vi "Render Recursive Partial with Wrong Key.vi"(8 "Error In":errorcluster) -> (0 "Error Out":errorcluster)   [LabVIEW 2018, in "Tests.lvlib" / "Render.lvlib"]
uses:
  Render.lvlib
  src/Toolkit/Data/Array/Array.lvclass
  D:/Users/cfield/Code/Field R&D Services/Labstache/src/Toolkit/Data/Datum/Datum.lvclass
  src/Toolkit/Data/Map/Map.lvclass
  src/Toolkit/Low-Level/Loaders/String/String.lvclass
  D:/Users/cfield/Code/Field R&D Services/Labstache/src/Toolkit/Low-Level/Loaders/Loader/Loader.lvclass
  src/Toolkit/Data/Pair/Support/From String.vi
  src/Toolkit/Data/Array/Support/From Strings.vi
  src/Toolkit/Data/Pair/Support/From Datum.vi
  src/Toolkit/Data/Map/Support/From Pair Array.vi
  src/Toolkit/Data/Array/Support/From Data.vi
  src/Toolkit/Low-Level/Renderer/Renderer.lvclass
  <vilib>/addons/_JKI Toolkits/Caraya/classes/Test/Test.lvclass
  <vilib>/addons/_JKI Toolkits/Caraya/classes/Assert/Assert.lvclass
  src/Toolkit/Data/Pair/Pair.lvclass
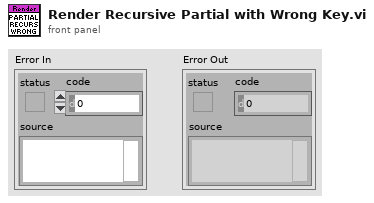
[diagram p1: front panel]
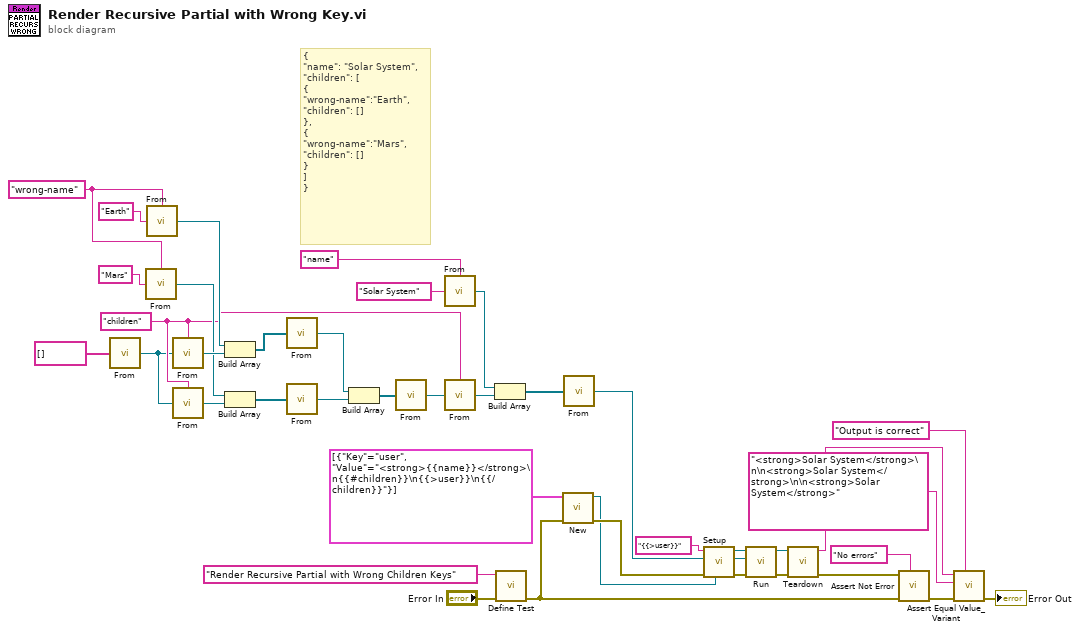
[diagram p0: block diagram]
diagram:
  w5 = "wrong-name" ("Key")
  w8 = "children" ("Key")
  # "{\n\"name\": \"Solar System\",\n\"children\": [\n{\n\"wrong-name\":\"Earth\",\n\"children\": []\n},\n{\n\"wrong-name\":\"Mars\",\n\"children\": []\n}\n]\n}"
  n1 = call-poly "From.vi"("Strings"=string[] []) -> ("Array"=w6:refnum<class "Array.lvclass">)  [unwired: 1 in]
  n2 = call-poly "From.vi"("Value"="Mars", "Key"=w5) -> ("Pair"=w13:refnum<class "Pair.lvclass">)
  n3 = call-poly "From.vi"("Value"="Earth", "Key"=w5) -> ("Pair"=w18:refnum<class "Pair.lvclass">)
  n4 = call-poly "From.vi"("Value"=w6, "Key"=w8) -> ("Pair"=w17:refnum<class "Pair.lvclass">)
  n5 = call-poly "From.vi"("Value"=w6, "Key"=w8) -> ("Pair"=w12:refnum<class "Pair.lvclass">)
  n6 = Build Array(w18, w17) -> (w16:refnum<class "Pair.lvclass">[])
  n7 = Build Array(w13, w12) -> (w11:refnum<class "Pair.lvclass">[])
  n8 = call-poly "From.vi"("Pairs"=w16) -> ("Map"=w15:refnum<class "Map.lvclass">)  [unwired: 1 in]
  n9 = call-poly "From.vi"("Pairs"=w11) -> ("Map"=w7:refnum<class "Map.lvclass">)  [unwired: 1 in]
  n10 = Build Array(w15, w7) -> (w23:refnum<class "Map.lvclass">[])
  n11 = call-poly "From.vi"("Data"=w23) -> ("Array"=w22:refnum<class "Array.lvclass">)  [unwired: 1 in]
  n12 = call-poly "From.vi"("Value"="Solar System", "Key"="name") -> ("Pair"=w21:refnum<class "Pair.lvclass">)
  n13 = call-poly "From.vi"("Value"=w22, "Key"=w8) -> ("Pair"=w20:refnum<class "Pair.lvclass">)
  n14 = Build Array(w21, w20) -> (w19:refnum<class "Pair.lvclass">[])
  n15 = call <vilib>:"Define Test.vi"("error in (no error)"="Error In", "Label (VI Title)"="Render Recursive Partial with Wrong Children Keys") -> ("error out"=w28:errorcluster)  [unwired: 9 in]
  n16 = call "New.vi"("Error In"=w28, "Key-Value Pairs"=cluster{"Key":string, "Value":string}[] [{"Key"="user", "Value"="<strong>{{name}}</strong>\n{{#children}}\n{{>user}}\n{{/children}}"}]) -> ("Error Out"=w30:errorcluster, "String"=w1:refnum<class "String.lvclass">)  [unwired: 8 in]
  n17 = call-poly "From.vi"("Pairs"=w19) -> ("Map"=w3:refnum<class "Map.lvclass">)  [unwired: 1 in]
  n18 = call "Setup.vi"("Loader"=w1, "Error In"=w30, "Data"=w3, "Value"="{{>user}}" ("format string")) -> ("Error Out"=w31:errorcluster, "Abstract Syntax Tree"=w2:refnum<class "Root.lvclass">, "Renderer"=w32:refnum<class "Renderer.lvclass">)  [unwired: 5 in]
  n19 = call-dynamic "Run.vi"("Error In"=w31, "Abstract Syntax Tree"=w2, "Renderer In"=w32) -> ("Error Out"=w33:errorcluster, "Renderer Out"=w4:refnum<class "Renderer.lvclass">)  [unwired: 7 in]
  n20 = call "Teardown.vi"("Error In"=w33, "Renderer"=w4) -> ("Error Out"=w35:errorcluster, "Output"=w34:string)  [unwired: 8 in]
  n21 = call <vilib>:"Assert Not Error.vi"("Label"="No errors", "error in (no error)"=w28, "Not Error?"=w35) -> ("error out"=w38:errorcluster)  [unwired: 8 in]
  n22 = call <vilib>:"Assert Equal Value_Variant.vi"("Label"="Output is correct", "error in (no error)"=w38, "Y"="<strong>Solar System</strong>\n\n<strong>Solar System</strong>\n\n<strong>Solar System</strong>", "X"=w34) -> ("error out"=→"Error Out":errorcluster)  [unwired: 7 in]
